vi "Begin.vi"(11 "Image Size":T1=enum."160x120") -> (0 "error out":errorcluster)   [LabVIEW 2011]
doc: "Called before other user functions, this VI is expected to open initial I/O refnums, load in file data, and do all program initialization. Notice that the <B>error out</B> terminal is simply used for data flow. Wiring it to other structures or subVIs ensures that this VI runs first."
uses:
  <vilib>/Rock Robotics/WPI/Camera/WPI_CameraImageSize.ctl
  <vilib>/Rock Robotics/WPI/Joystick/WPI_JoystickDeviceEnum.ctl
  <vilib>/Rock Robotics/WPI/Camera/WPI_CameraWhite Balance Values.ctl
  <vilib>/Rock Robotics/WPI/Camera/WPI_CameraExposure Values.ctl
  <vilib>/Rock Robotics/WPI/Camera/WPI_CameraFrameRate.ctl
  <vilib>/Rock Robotics/SystemInterfaces/DIO/FPGA_DIOPWMChannel.ctl
  <vilib>/Rock Robotics/SystemInterfaces/Typedef/FPGA_TypedefDigitalModule.ctl
  <vilib>/Rock Robotics/SystemInterfaces/DIO/FPGA_DIOChannel.ctl
  <vilib>/Rock Robotics/WPI/Encoder/WPI_EncoderType.ctl
  <vilib>/Rock Robotics/SystemInterfaces/AI/FPGA_AIChannel.ctl
  <vilib>/Rock Robotics/SystemInterfaces/Typedef/FPGA_TypedefAnalogModule.ctl
  <vilib>/Rock Robotics/WPI/MotorControl/WPI_MotorControlOpen Victor.vi
  <vilib>/Rock Robotics/WPI/Counter/WPI_CounterDigitalInputToDigitalSource.vi
panel:
  in  "Invert Direction (False) 2":bool
  in  "Invert Direction (False)":bool
  in  "Invert 8":bool
  in  "Invert 7":bool
  in  "Invert 6":bool
  in  "Invert 5":bool
  in  "Invert 4":bool
  in  "Invert 3":bool
  in  "Invert 2":bool
  in  "Invert":bool
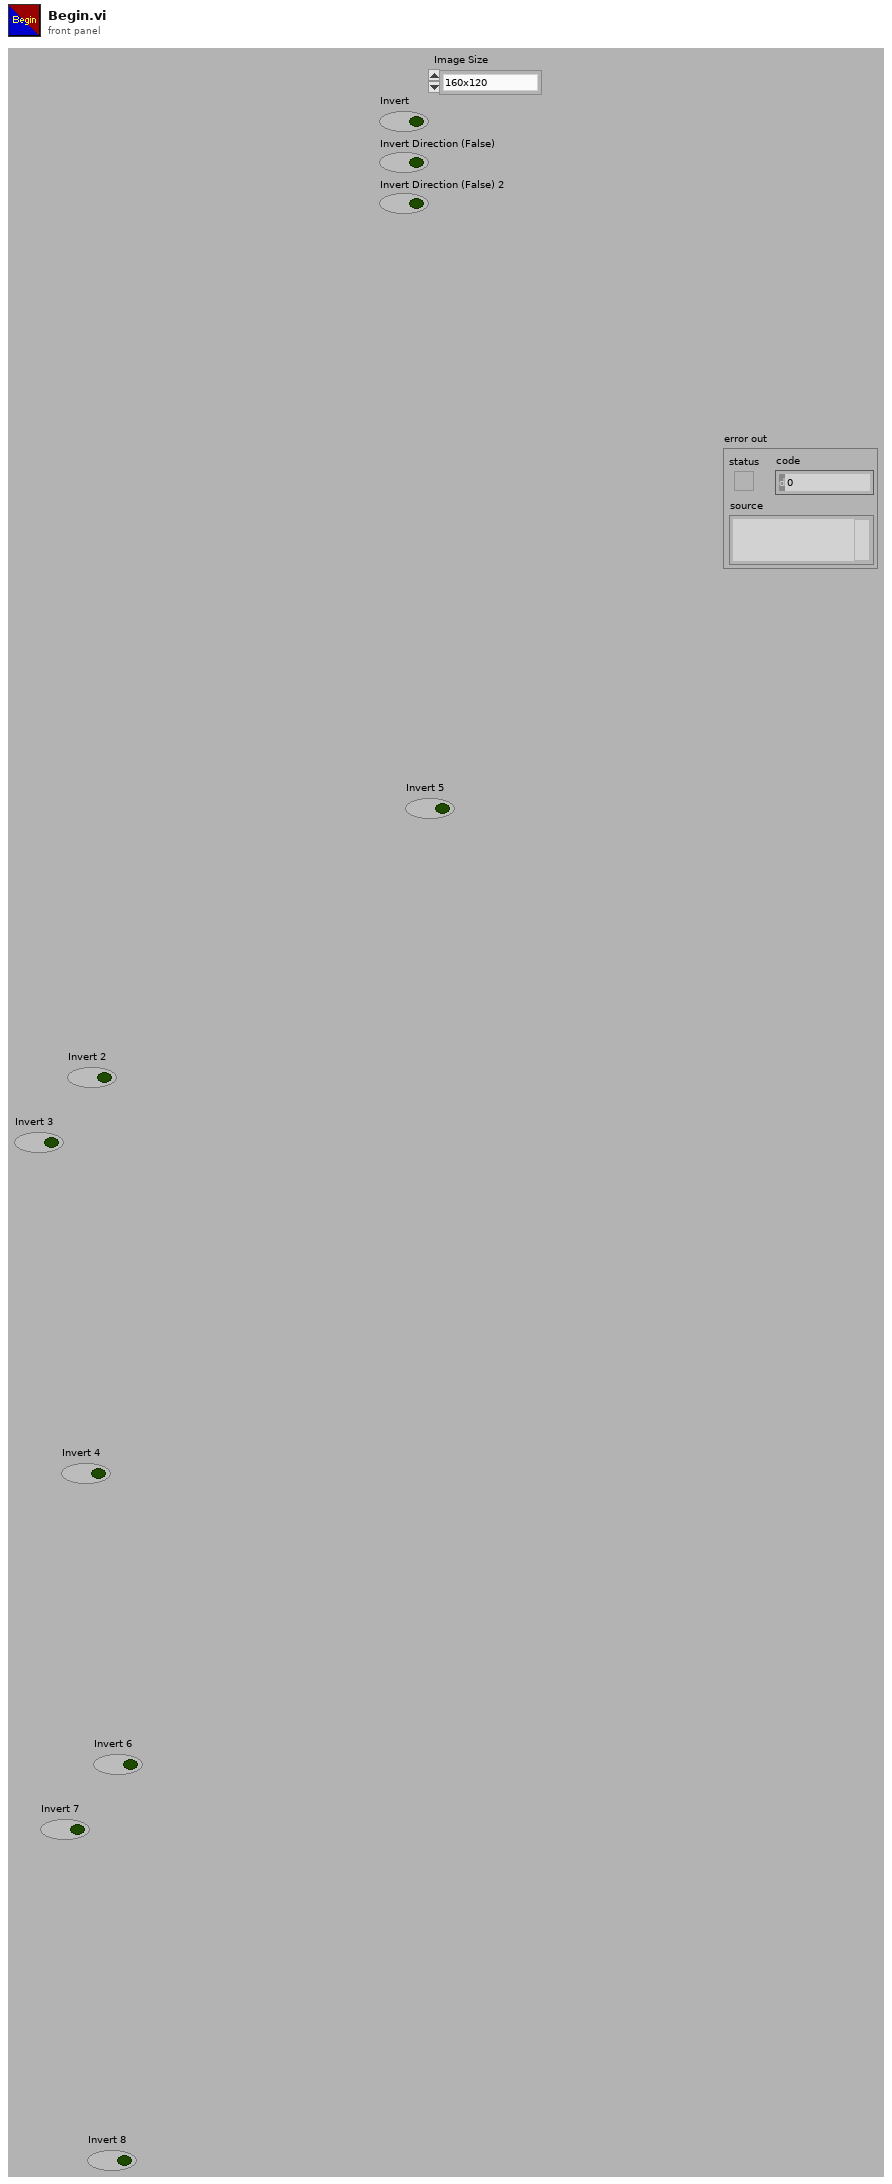
[diagram p1: front panel]
types:
  T1 = typedef "WPI_CameraImageSize.ctl" = enum16{"640x480", "320x240", "160x120"}
  T2 = typedef "FPGA_AIChannel.ctl" = enum8{"AI 1", "AI 2", "AI 3", "AI 4", "AI 5", "AI 6", "AI 7", "AI 8", "Invalid"}
  T3 = typedef "FPGA_TypedefAnalogModule.ctl" = enum16{"Analog Module 1", "Analog Module 2"}
  T4 = typedef "WPI_EncoderType.ctl" = enum16{"1x", "2x", "4x"}
  T5 = typedef "FPGA_DIOChannel.ctl" = enum8{"DIO 1", "DIO 2", "DIO 3", "DIO 4", "DIO 5", "DIO 6", "DIO 7", "DIO 8", "DIO 9", "DIO 10", "DIO 11", "DIO 12", "DIO 13", "DIO 14", "Invalid"}
  T6 = typedef "FPGA_TypedefDigitalModule.ctl" = enum16{"Digital Module 1", "Digital Module 2"}
  T7 = typedef "FPGA_DIOPWMChannel.ctl" = enum8{"PWM 1", "PWM 2", "PWM 3", "PWM 4", "PWM 5", "PWM 6", "PWM 7", "PWM 8", "PWM 9", "PWM 10", "Invalid"}
  T8 = typedef "WPI_JoystickDeviceEnum.ctl" = enum16{"USB 1", "USB 2", "USB 3", "USB 4", "Kinect 1", "Kinect 2"}
  T9 = typedef "WPI_CameraFrameRate.ctl" = u32
  T10 = typedef "WPI_CameraExposure Values.ctl" = enum16{"Auto", "Flicker-free 50 Hz", "Flicker-free 60 Hz", "Hold current"}
  T11 = typedef "WPI_CameraWhite Balance Values.ctl" = enum16{"Auto", "Fixed indoor", "Fixed outdoor 1", "Fixed outdoor 2", "Fixed fluorescent 1", "Fixed fluorescent 2", "Hold current"}
  T12 = typedef "WPI_MotorControlDeviceRef.ctl" = cluster{"DeviceStatus":errorcluster, "Type":enum16{"PWM", "CAN"}, "PWM":cluster{"Digital Module":T6, "PWM Channel":T7, "DeadBand":T13}, "CAN":cluster{"Device Number":u8, "Control Mode":T14, "Semaphore":T15, "Max Vout":dbl}, "Invert":bool, "TransformRef":T16, "InvTransformRef":T16}
  T13 = typedef "WPI_PWMDeadband.ctl" = cluster{"Name":string, "maxPositivePwm":i32, "minPositivePwm":i32, "centerPwm":i32, "maxNegativePwm":i32, "minNegativePwm":i32, "angularRange":u16}
  T14 = typedef "WPI_CANJaguar_ControlMode.ctl" = enum8{"Percent VBus", "Current", "Speed", "Position", "Voltage"}
  T15 = typedef "Semaphore RefNum" = refnum<k1>
  T16 = typedef "WPI_PWMTransform_ConPane.ctl" = refnum<vi>
  T17 = typedef "WPI_JoystickDevRef.ctl" = cluster{"Device":T8}
  T18 = typedef "WPI_CameraDevRef.ctl" = cluster{"Camera Address":string, "CameraStatus":errorcluster, "Acquire Image Notifier":refnum<notifier>}
  T19 = typedef "WPI_DigitalInputDevRef.ctl" = cluster{"DevStatus":errorcluster, "DIO Channel":T5, "Digital Module":T6}
  T20 = typedef "FPGA_CounterEncoderSourceConvertionLVSourceType.ctl" = cluster{"DevStatus":errorcluster, "AnalogTriggerMode?":bool, "DigitalMode":cluster{"Digital Module":T6, "DIO Channel":T21}, "AnalogTriggerMode":cluster{"AnalogTriggerIndex":T22, "OutputType":T23}}
  T21 = typedef "FPGA_DIODigitalSourceChannel.ctl" = enum8{"DIO 1", "DIO 2", "DIO 3", "DIO 4", "DIO 5", "DIO 6", "DIO 7", "DIO 8", "DIO 9", "DIO 10", "DIO 11", "DIO 12", "DIO 13", "DIO 14", "Disabled"}
  T22 = typedef "FPGA_AnalogTriggerIndex.ctl" = enum8{"Trig 0", "Trig 1", "Trig 2", "Trig 3", "Trig 4", "Trig 5", "Trig 6", "Trig 7", "Invalid"}
  T23 = typedef "FPGA_AnalogTriggerOutType.ctl" = enum16{"InWindow", "TriggerState", "Rising", "Falling"}
  T24 = typedef "WPI_EncoderDevRef.ctl" = cluster{"DevStatus":errorcluster, "EncoderIndex":T25, "CounterIndex":T26, "DistancePerCount":dbl, "Decoding Type":T4}
  T25 = typedef "FPGA_EncoderIdx.ctl" = enum8{"Enc 0", "Enc 1", "Enc 2", "Enc 3", "Invalid"}
  T26 = typedef "FPGA_CounterCtrSystemIndex.ctl" = enum8{"Ctr 0", "Ctr 1", "Ctr 2", "Ctr 3", "Ctr 4", "Ctr 5", "Ctr 6", "Ctr 7", "Invalid"}
  T27 = typedef "WPI_AnalogChannelDevRef.ctl" = cluster{"DevStatus":errorcluster, "Analog Module":T3, "Analog Channel":T2}
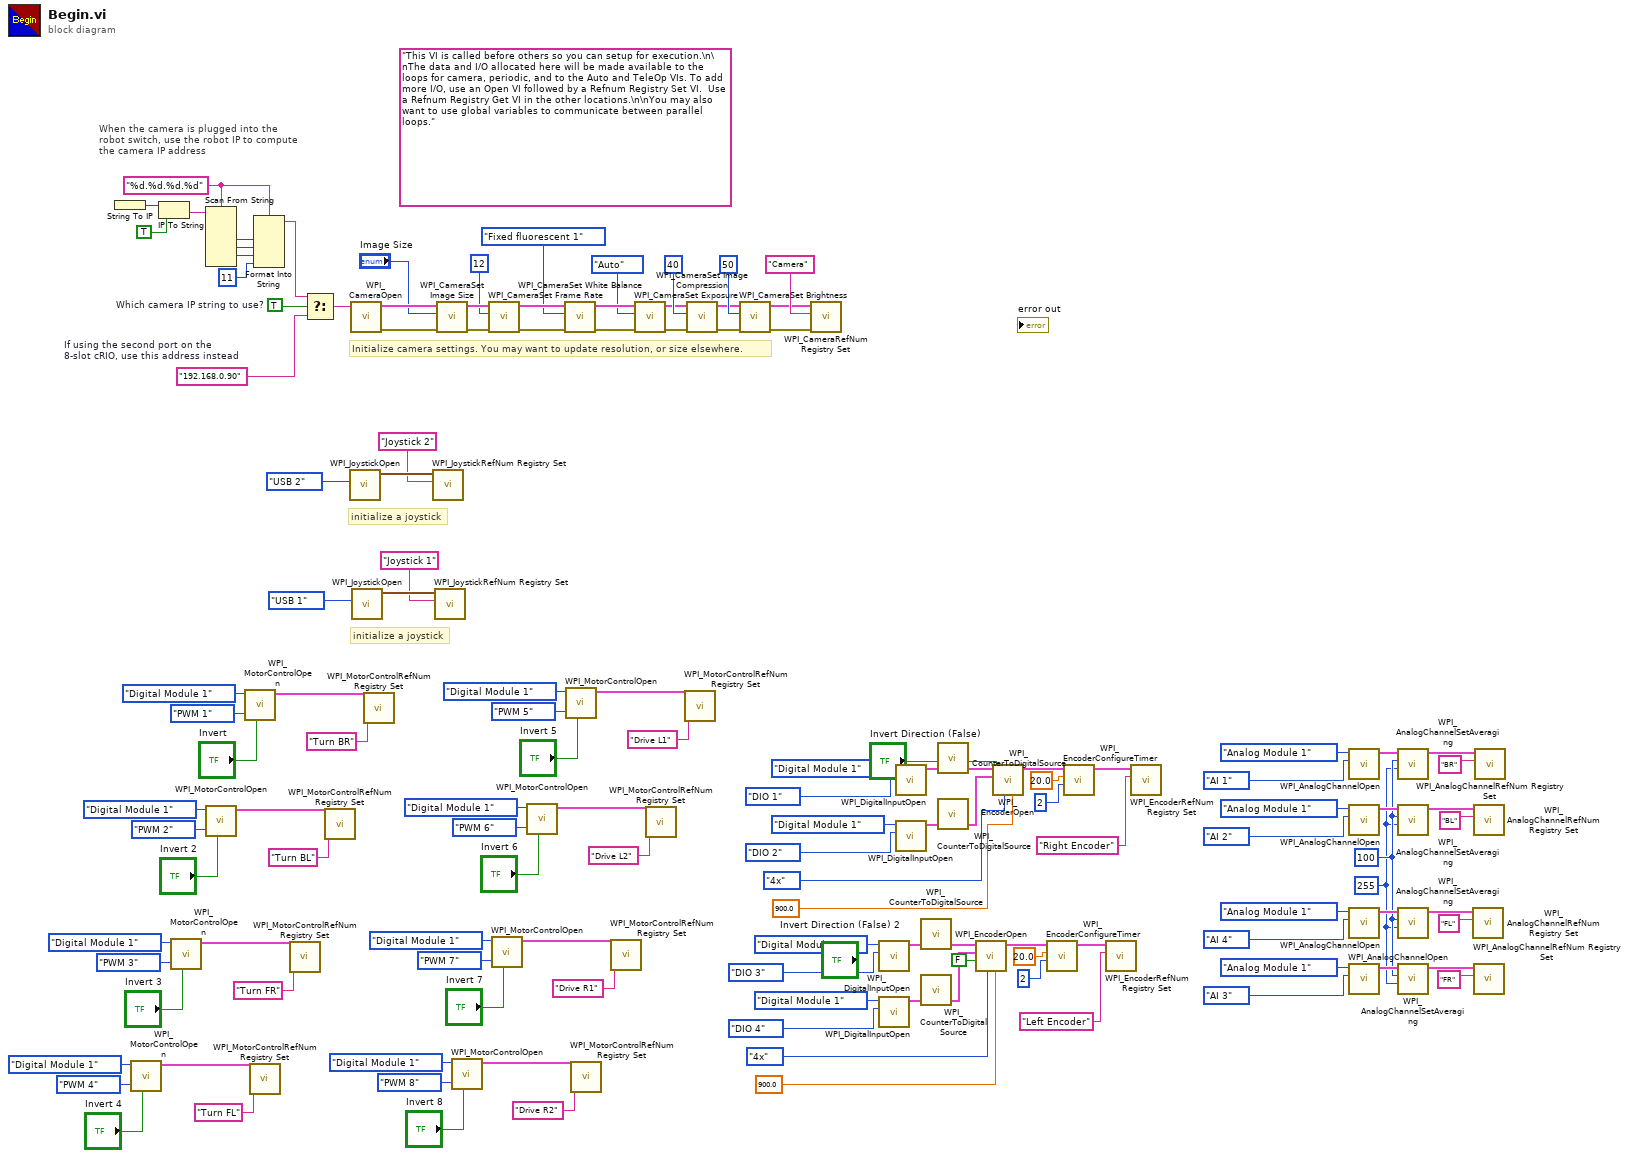
[diagram p0: block diagram]
diagram:
  w1 = u8 255 ("OversampleBits")
  w2 = u8 100 ("AverageBits")
  w98 = TRUE  # Which camera IP string to use?
  w102 = "%d.%d.%d.%d" ("format string")
  (unwired) "This VI is called before others so you can setup for execution.\n\nThe data and I/O allocated here will be made available to the loops for camera, periodic, and to the Auto and TeleOp VIs. To add more I/O, use an Open VI followed by a Refnum Registry Set VI.  Use a Refnum Registry Get VI in the other locations.\n\nYou may also want to use global variables to communicate between parallel loops."
  w99 = "192.168.0.90"  # If using the second port on the 8-slot cRIO, use this address instead
  # "initialize a joystick"
  # "When the camera is plugged into the\nrobot switch, use the robot IP to compute\nthe camera IP address"
  # "initialize a joystick"
  # "Initialize camera settings. You may want to update resolution, or size elsewhere."
  n1 = String To IP() -> (0:w109:u32)  [unwired: 1 in]
  n2 = call-poly <vilib>:"WPI_MotorControlOpen.vi"("Invert"="Invert 4", "PWM Channel"=FPGA_DIOPWMChannel."PWM 4", "Digital Module (Module 1)"=FPGA_TypedefDigitalModule."Digital Module 1") -> ("MotorControlDeviceRef"=w82:T12)  [unwired: 7 in, 1 out]
  n3 = IP To String(1:TRUE ("dot notation? (F)"), 2:w109) -> (0:w107:string)
  n4 = call-poly <vilib>:"WPI_MotorControlOpen.vi"("Invert"="Invert 3", "PWM Channel"=FPGA_DIOPWMChannel."PWM 3", "Digital Module (Module 1)"=FPGA_TypedefDigitalModule."Digital Module 1") -> ("MotorControlDeviceRef"=w86:T12)  [unwired: 7 in, 1 out]
  n5 = Scan From String(format string=w102, input string=w107) -> (output 1=w106:i32, output 2=w105:i32, output 3=w104:i32)  [unwired: 7 in, 3 out]
  n6 = call-poly <vilib>:"WPI_MotorControlOpen.vi"("Invert"="Invert 2", "PWM Channel"=FPGA_DIOPWMChannel."PWM 2", "Digital Module (Module 1)"=FPGA_TypedefDigitalModule."Digital Module 1") -> ("MotorControlDeviceRef"=w90:T12)  [unwired: 7 in, 1 out]
  n7 = call-poly <vilib>:"WPI_MotorControlOpen.vi"("Invert"="Invert", "PWM Channel"=FPGA_DIOPWMChannel."PWM 1", "Digital Module (Module 1)"=FPGA_TypedefDigitalModule."Digital Module 1") -> ("MotorControlDeviceRef"=w94:T12)  [unwired: 7 in, 1 out]
  n8 = call <vilib>:"WPI_MotorControlRefNum Registry Set.vi"("refnum name"="Turn FL", "MotorControlDevRef"=w82) -> ()  [unwired: 8 in, 2 out]
  n9 = Format Into String(format string=w102, w106, w105, w104, 11 ("Compression")) -> (resulting string=w100:string)  [unwired: 2 in, 1 out]
  n10 = call <vilib>:"WPI_MotorControlRefNum Registry Set.vi"("refnum name"="Turn FR", "MotorControlDevRef"=w86) -> ()  [unwired: 8 in, 2 out]
  n11 = Select(t=w100, s=w98, f=w99) -> (s? t:f=w101:string)
  n12 = call <vilib>:"WPI_MotorControlRefNum Registry Set.vi"("refnum name"="Turn BL", "MotorControlDevRef"=w90) -> ()  [unwired: 8 in, 2 out]
  n13 = call <vilib>:"WPI_JoystickOpen.vi"("JoystickDevice"=WPI_JoystickDeviceEnum."USB 2") -> ("JoystickDevRef"=w97:T17)  [unwired: 10 out]
  n14 = call <vilib>:"WPI_CameraOpen.vi"("Camera Address"=w101) -> ("error out"=w122:errorcluster, "CameraDevRef"=w123:T18)  [unwired: 1 in, 8 out]
  n15 = call <vilib>:"WPI_JoystickOpen.vi"("JoystickDevice"=WPI_JoystickDeviceEnum."USB 1") -> ("JoystickDevRef"=w132:T17)  [unwired: 10 out]
  n16 = call <vilib>:"WPI_MotorControlRefNum Registry Set.vi"("refnum name"="Turn BR", "MotorControlDevRef"=w94) -> ()  [unwired: 8 in, 2 out]
  n17 = call <vilib>:"WPI_JoystickRefNum Registry Set.vi"("refnum name"="Joystick 2", "JoystickDevRef"=w97) -> ()  [unwired: 1 in, 9 out]
  n18 = call <vilib>:"WPI_JoystickRefNum Registry Set.vi"("refnum name"="Joystick 1", "JoystickDevRef"=w132) -> ()  [unwired: 1 in, 9 out]
  n19 = call <vilib>:"WPI_CameraSet Image Size.vi"("error in (no error)"=w122, "Image Size"="Image Size", "CameraDevRef"=w123) -> ("error out"=w121:errorcluster, "CameraDevRef Out"=w124:T18)  [unwired: 7 out]
  n20 = call-poly <vilib>:"WPI_MotorControlOpen.vi"("Invert"="Invert 8", "PWM Channel"=FPGA_DIOPWMChannel."PWM 8", "Digital Module (Module 1)"=FPGA_TypedefDigitalModule."Digital Module 1") -> ("MotorControlDeviceRef"=w62:T12)  [unwired: 7 in, 1 out]
  n21 = call <vilib>:"WPI_CameraSet Frame Rate.vi"("error in (no error)"=w121, "Frame Rate (fps)"=T9 12, "CameraDevRef"=w124) -> ("error out"=w120:errorcluster, "CameraDevRef Out"=w126:T18)  [unwired: 7 out]
  n22 = call-poly <vilib>:"WPI_MotorControlOpen.vi"("Invert"="Invert 7", "PWM Channel"=FPGA_DIOPWMChannel."PWM 7", "Digital Module (Module 1)"=FPGA_TypedefDigitalModule."Digital Module 1") -> ("MotorControlDeviceRef"=w66:T12)  [unwired: 7 in, 1 out]
  n23 = call-poly <vilib>:"WPI_MotorControlOpen.vi"("Invert"="Invert 6", "PWM Channel"=FPGA_DIOPWMChannel."PWM 6", "Digital Module (Module 1)"=FPGA_TypedefDigitalModule."Digital Module 1") -> ("MotorControlDeviceRef"=w70:T12)  [unwired: 7 in, 1 out]
  n24 = call <vilib>:"WPI_CameraSet White Balance.vi"("error in (no error)"=w120, "White Balance"=WPI_CameraWhite_Balance_Values."Fixed fluorescent 1", "CameraDevRef"=w126) -> ("error out"=w119:errorcluster, "CameraDevRef Out"=w125:T18)  [unwired: 7 out]
  n25 = call-poly <vilib>:"WPI_MotorControlOpen.vi"("Invert"="Invert 5", "PWM Channel"=FPGA_DIOPWMChannel."PWM 5", "Digital Module (Module 1)"=FPGA_TypedefDigitalModule."Digital Module 1") -> ("MotorControlDeviceRef"=w74:T12)  [unwired: 7 in, 1 out]
  n26 = call <vilib>:"WPI_MotorControlRefNum Registry Set.vi"("refnum name"="Drive R2", "MotorControlDevRef"=w62) -> ()  [unwired: 8 in, 2 out]
  n27 = call <vilib>:"WPI_MotorControlRefNum Registry Set.vi"("refnum name"="Drive R1", "MotorControlDevRef"=w66) -> ()  [unwired: 8 in, 2 out]
  n28 = call <vilib>:"WPI_CameraSet Exposure.vi"("error in (no error)"=w119, "Exposure"=WPI_CameraExposure_Values."Auto", "CameraDevRef"=w125) -> ("error out"=w118:errorcluster, "CameraDevRef Out"=w128:T18)  [unwired: 7 out]
  n29 = call <vilib>:"WPI_MotorControlRefNum Registry Set.vi"("refnum name"="Drive L2", "MotorControlDevRef"=w70) -> ()  [unwired: 8 in, 2 out]
  n30 = call <vilib>:"WPI_MotorControlRefNum Registry Set.vi"("refnum name"="Drive L1", "MotorControlDevRef"=w74) -> ()  [unwired: 8 in, 2 out]
  n31 = call <vilib>:"WPI_CameraSet Image Compression.vi"("error in (no error)"=w118, "Compression"=40, "CameraDevRef"=w128) -> ("error out"=w117:errorcluster, "CameraDevRef Out"=w127:T18)  [unwired: 7 out]
  n32 = call <vilib>:"WPI_CameraSet Brightness.vi"("error in (no error)"=w117, "Brightness"=50, "CameraDevRef"=w127) -> ("error out"=w115:errorcluster, "CameraDevRef Out"=w116:T18)  [unwired: 7 out]
  n33 = call <vilib>:"WPI_CameraRefNum Registry Set.vi"("error in (no error)"=w115, "refnum name"="Camera", "CameraDevRef"=w116) -> ()  [unwired: 9 out]
  n34 = call <vilib>:"WPI_DigitalInputOpen.vi"("DIO Channel"=FPGA_DIOChannel."DIO 3", "Digital Module (Module 1)"=FPGA_TypedefDigitalModule."Digital Module 1") -> ("DigitalInputDevRef"=w43:T19)  [unwired: 8 in, 1 out]
  n35 = call <vilib>:"WPI_DigitalInputOpen.vi"("DIO Channel"=FPGA_DIOChannel."DIO 4", "Digital Module (Module 1)"=FPGA_TypedefDigitalModule."Digital Module 1") -> ("DigitalInputDevRef"=w44:T19)  [unwired: 8 in, 1 out]
  n36 = call <vilib>:"WPI_DigitalInputOpen.vi"("DIO Channel"=FPGA_DIOChannel."DIO 1", "Digital Module (Module 1)"=FPGA_TypedefDigitalModule."Digital Module 1") -> ("DigitalInputDevRef"=w50:T19)  [unwired: 8 in, 1 out]
  n37 = call <vilib>:"WPI_DigitalInputOpen.vi"("DIO Channel"=FPGA_DIOChannel."DIO 2", "Digital Module (Module 1)"=FPGA_TypedefDigitalModule."Digital Module 1") -> ("DigitalInputDevRef"=w52:T19)  [unwired: 8 in, 1 out]
  n38 = call-poly <vilib>:"WPI_CounterToDigitalSource.vi"("DigitalInputDevRef"=w43) -> ("Digital Source"=w38:T20)  [unwired: 6 in]
  n39 = call-poly <vilib>:"WPI_CounterToDigitalSource.vi"("DigitalInputDevRef"=w44) -> ("Digital Source"=w37:T20)  [unwired: 6 in]
  n40 = call-poly <vilib>:"WPI_CounterToDigitalSource.vi"("DigitalInputDevRef"=w50) -> ("Digital Source"=w49:T20)  [unwired: 6 in]
  n41 = call-poly <vilib>:"WPI_CounterToDigitalSource.vi"("DigitalInputDevRef"=w52) -> ("Digital Source"=w51:T20)  [unwired: 6 in]
  n42 = call <vilib>:"WPI_EncoderOpen.vi"("DistancePerCount"=900.0, "Decoding Type"=WPI_EncoderType."4x", "Invert Direction (False)"=FALSE, "BSource"=w37, "ASource"=w38) -> ("EncoderDevRef"=w36:T24)  [unwired: 5 in, 1 out]
  n43 = call <vilib>:"WPI_EncoderOpen.vi"("DistancePerCount"=900.0, "Decoding Type"=WPI_EncoderType."4x", "Invert Direction (False)"="Invert Direction (False)", "BSource"=w51, "ASource"=w49) -> ("EncoderDevRef"=w34:T24)  [unwired: 5 in, 1 out]
  n44 = call <vilib>:"WPI_EncoderConfigureTimer.vi"("Number Samples to Average"=u8 2, "Minimum Rate"=20.0, "EncoderDevRef"=w36) -> ("EncoderDevRef"=w35:T24)  [unwired: 7 in, 1 out]
  n45 = call <vilib>:"WPI_EncoderConfigureTimer.vi"("Number Samples to Average"=u8 2, "Minimum Rate"=20.0, "EncoderDevRef"=w34) -> ("EncoderDevRef"=w33:T24)  [unwired: 7 in, 1 out]
  n46 = call <vilib>:"WPI_EncoderRefNum Registry Set.vi"("refnum name"="Left Encoder", "EncoderDevRef"=w35) -> ()  [unwired: 8 in, 2 out]
  n47 = call <vilib>:"WPI_EncoderRefNum Registry Set.vi"("refnum name"="Right Encoder", "EncoderDevRef"=w33) -> ()  [unwired: 8 in, 2 out]
  n48 = call <vilib>:"WPI_AnalogChannelOpen.vi"("Analog Channel"=FPGA_AIChannel."AI 1", "Analog Module (Module 1)"=FPGA_TypedefAnalogModule."Analog Module 1") -> ("AIDeviceRef"=w15:T27)  [unwired: 8 in, 1 out]
  n49 = call <vilib>:"WPI_AnalogChannelOpen.vi"("Analog Channel"=FPGA_AIChannel."AI 2", "Analog Module (Module 1)"=FPGA_TypedefAnalogModule."Analog Module 1") -> ("AIDeviceRef"=w20:T27)  [unwired: 8 in, 1 out]
  n50 = call <vilib>:"WPI_AnalogChannelOpen.vi"("Analog Channel"=FPGA_AIChannel."AI 4", "Analog Module (Module 1)"=FPGA_TypedefAnalogModule."Analog Module 1") -> ("AIDeviceRef"=w10:T27)  [unwired: 8 in, 1 out]
  n51 = call <vilib>:"WPI_AnalogChannelOpen.vi"("Analog Channel"=FPGA_AIChannel."AI 3", "Analog Module (Module 1)"=FPGA_TypedefAnalogModule."Analog Module 1") -> ("AIDeviceRef"=w5:T27)  [unwired: 8 in, 1 out]
  n52 = call <vilib>:"WPI_AnalogChannelSetAveraging.vi"("OversampleBits"=w1, "AverageBits"=w2, "AIDeviceRef"=w15) -> ("AIDeviceRef"=w14:T27)  [unwired: 7 in, 1 out]
  n53 = call <vilib>:"WPI_AnalogChannelSetAveraging.vi"("OversampleBits"=w1, "AverageBits"=w2, "AIDeviceRef"=w20) -> ("AIDeviceRef"=w19:T27)  [unwired: 7 in, 1 out]
  n54 = call <vilib>:"WPI_AnalogChannelSetAveraging.vi"("OversampleBits"=w1, "AverageBits"=w2, "AIDeviceRef"=w10) -> ("AIDeviceRef"=w9:T27)  [unwired: 7 in, 1 out]
  n55 = call <vilib>:"WPI_AnalogChannelSetAveraging.vi"("OversampleBits"=w1, "AverageBits"=w2, "AIDeviceRef"=w5) -> ("AIDeviceRef"=w4:T27)  [unwired: 7 in, 1 out]
  n56 = call <vilib>:"WPI_AnalogChannelRefNum Registry Set.vi"("refnum name"="FL", "AIDeviceRef"=w9) -> ()  [unwired: 8 in, 2 out]
  n57 = call <vilib>:"WPI_AnalogChannelRefNum Registry Set.vi"("refnum name"="BL", "AIDeviceRef"=w19) -> ()  [unwired: 8 in, 2 out]
  n58 = call <vilib>:"WPI_AnalogChannelRefNum Registry Set.vi"("refnum name"="FR", "AIDeviceRef"=w4) -> ()  [unwired: 8 in, 2 out]
  n59 = call <vilib>:"WPI_AnalogChannelRefNum Registry Set.vi"("refnum name"="BR", "AIDeviceRef"=w14) -> ()  [unwired: 8 in, 2 out]
